vi "Send Command.vi"(7 "Config offset":u64 format="%x", 8 "error in (no error)":errorcluster, 9 "Command payload":u64 format="%x", 10 "Command number":T1, 11 "RP Communicator in":refnum<class "RP Communicator.lvclass">) -> (0 "error out":errorcluster, 3 "RP Communicator out":refnum<class "RP Communicator.lvclass">)   [LabVIEW 2018, in "RP Communicator.lvclass"]
uses:
  RP Communicator.lvclass
  RP Command.ctl
  RP Communicator.lvclass/RP Communicator.ctl
  Read Timeout.vi
  RP Write Command TCP.vi
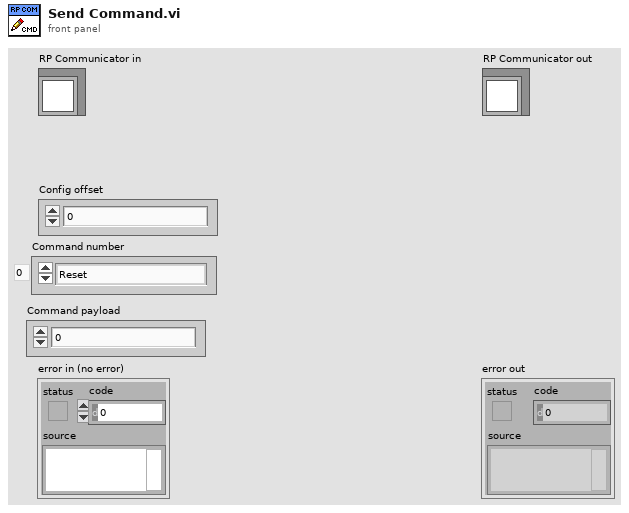
[diagram p1: front panel]
types:
  T1 = typedef "RP Command.ctl" = enum16{"Reset", "Read IDN", "Stop server", "Get status", "Get temperature", "Connect client", "Arm", "Software trigger", "Get whole buffer", "Get chunk", "System call", "Get config", "Set config", "Recieve data", "Recieve Calibartion", "Transmit data"}
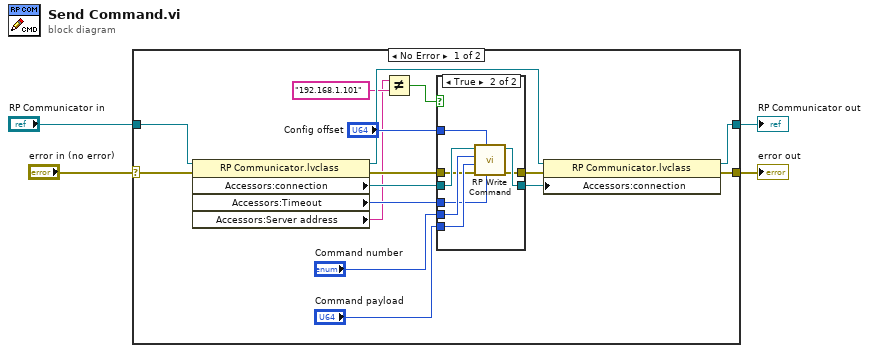
[diagram p0: block diagram]
diagram:
  n1 = case shown="No Error" "error in (no error)" {
    selector: "error in (no error)" -> [w12 w32]
    tunnel: [w9 w32] -> w3
    tunnel: [w14 w31] -> w1
    tunnel: "RP Communicator in" -> [w16 w31]
    frame No Error {
      n2 = property class="RP Communicator.lvclass"(reference=w16, error in=w12) -> (reference out=w15:refnum<class "RP Communicator.lvclass">, error out=w11:errorcluster, "Accessors:connection"=w20:refnum<k5>, "Accessors:Timeout"=w8:i32, "Accessors:Server address"=w6:string)
      n3 = Not Equal?(x=w6, y="192.168.1.101") -> (x != y?=w5:bool)
      n4 = case shown="True" w5 {
        tunnel: w20 -> [w21 w30]
        tunnel: "Config offset" -> [_ w29]
        tunnel: "Command number" -> [_ w28]
        tunnel: "Command payload" -> [_ w27]
        tunnel: [w21 w26] -> w13
        tunnel: w11 -> [w22 w25]
        tunnel: [w22 w24] -> w10
        tunnel: w8 -> [_ w23]
        frame False {
        }
        frame True {
          n5 = call-poly "RP Write Command.vi"("timeout ms (25000)"=w23, "Config offset"=w29, "Error In"=w25, "Command payload"=w27, "Command number"=w28, "connection ID"=w30) -> ("Error Out"=w24:errorcluster, "connection ID out"=w26:refnum<k5>)  [unwired: 3 in, 1 out]
        }
      }
      n6 = property class="RP Communicator.lvclass"(reference=w15, error in=w10, "Accessors:connection"=w13) -> (reference out=w14:refnum<class "RP Communicator.lvclass">, error out=w9:errorcluster)
    }
    frame Error {
    }
  }
  "error out" <- w3
  "RP Communicator out" <- w1
